vi "_RT_CtrlLoop_DigitalAnalogueInput.vi"(6 "ExpVar in":refnum<class "ExpVar.lvclass">, 8 "error in (no error)":errorcluster) -> ()   [LabVIEW 2018]
uses:
  PublicSubVI/NewExpVar/ExpVar.lvclass
  PublicSubVI/Ctl/_ctl_RT_extDO.ctl
  PublicSubVI/Ctl/_ctl_RT_FPGA_Function.ctl
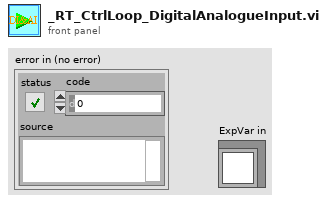
[diagram p1: front panel]
types:
  T1 = enum16{"None", "D999", "ExtAO", "ExtDO", "ExtDI_Label", "Signal_Remarks", "Script"}
  T2 = typedef "_ctl_RT_extDO.ctl" = cluster{"Label":string, "Boolean":bool}[]
  T3 = enum16{"via string label", "Laser", "Pressure", "TMP", "Script", "Signal Remarks", "ExtAO", "ExtDO", "ExtDI", "D999"}
  T4 = typedef "_ctl_RT_FPGA_Function.ctl" = enum16{"Initialisation", "Execution", "Digital In"}
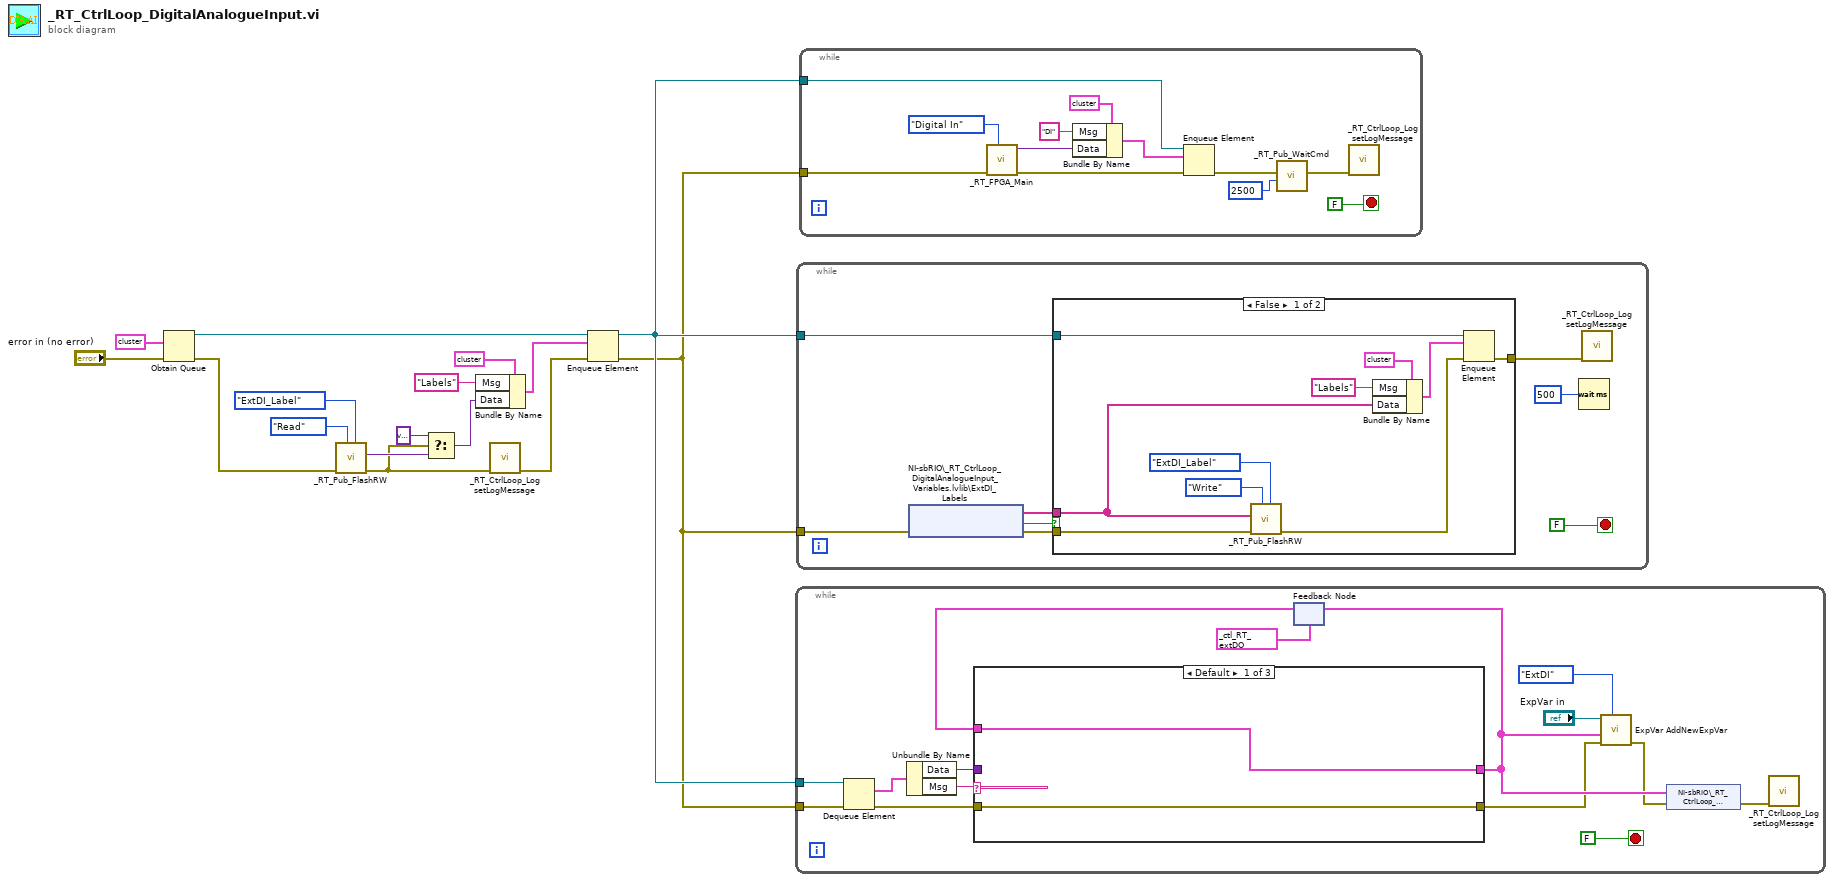
[diagram p0: block diagram]
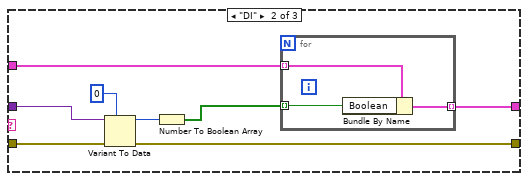
[diagram p2: hidden frame]
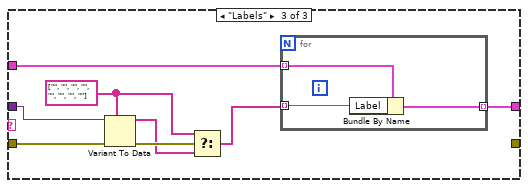
[diagram p3: hidden frame]
diagram:
  n1 = Obtain Queue(element data type=cluster{"Data":variant, "Msg":string} {"Data"=variant, "Msg"=""}, error in (no error)="error in (no error)") -> (queue out=w15:refnum<queue>, error out=w7:errorcluster)  [unwired: 3 in, 1 out]
  n2 = call "_RT_Pub_FlashRW.vi"("FileEnum"=T1."ExtDI_Label", "State"=enum16{"Read", "Write"}."Read", "error in (no error)"=w7) -> ("error out"=w2:errorcluster, "Value"=w5:variant)  [unwired: 6 in, 1 out]
  n3 = Select(t=variant, s=w2, f=w5) -> (s? t:f=w3:variant)
  n4 = Bundle By Name(cluster=cluster{"Data":variant, "Msg":string} {"Data"=variant, "Msg"=""}, "Msg"="Labels", "Data"=w3) -> (w13:cluster{"Data":variant, "Msg":string})
  n5 = call "_RT_CtrlLoop_Log setLogMessage.vi"("error in"=w2) -> ("error out"=w1:errorcluster)  [unwired: 9 in, 1 out]
  n6 = Enqueue Element(queue=w15, element=w13, error in (no error)=w1) -> (queue out=w11:refnum<queue>, error out=w10:errorcluster)  [unwired: 1 in, 1 out]
  n7 = while {
    tunnel: w11 -> [w31]
    tunnel: w10 -> [w30]
    stop <- FALSE stop-if-true
    n8 = Dequeue Element(queue=w31, error in (no error)=w30) -> (element=w19:cluster{"Data":variant, "Msg":string}, error out=w27:errorcluster)  [unwired: 1 in, 2 out]
    n9 = Unbundle By Name(w19) -> ("Data"=w28:variant, "Msg"=w29:string)
    n10 = feedback #1(T2 [{"Label"="", "Boolean"=FALSE}, {"Label"="", "Boolean"=FALSE}, {"Label"="", "Boolean"=FALSE}, {"Label"="", "Boolean"=FALSE}, {"Label"="", "Boolean"=FALSE}, {"Label"="", "Boolean"=FALSE}, {"Label"="", "Boolean"=FALSE}, {"Label"="", "Boolean"=FALSE}] ("DI in")) -> (w25:T2)
    n11 = case shown="Default" w29 {
      tunnel: w28 -> [_ w40 w52]
      tunnel: w27 -> [w32 w39 w51]
      tunnel: w25 -> [w33 w37 w50]
      tunnel: [w33 w35 w49] -> w22
      tunnel: [w32 w34 _] -> w21
      frame Default {
      }
      frame "DI" {
        n12 = Variant To Data(error in=w39, type=u8 0, Variant=w40) -> (data=w38:u8, error out=w34:errorcluster)
        n13 = Number To Boolean Array(number=w38) -> (Boolean array=w36:bool[])
        n14 = for {
          tunnel: w37 -> [w44] mode=indexing
          tunnel: w36 -> [w43] mode=indexing
          tunnel: [w42] -> w35 mode=indexing
          n15 = Bundle By Name(cluster=w44, "Boolean"=w43) -> (w42:cluster{"Label":string, "Boolean":bool})
        }
      }
      frame "Labels" {
        w46 = string[] ["", "", "", "", "", "", "", ""]
        n16 = Variant To Data(error in=w51, type=w46, Variant=w52) -> (data=w47:string[], error out=w48:errorcluster)
        n17 = Select(t=w46, s=w48, f=w47) -> (s? t:f=w45:string[])
        n18 = for {
          tunnel: w50 -> [w55] mode=indexing
          tunnel: w45 -> [w54] mode=indexing
          tunnel: [w53] -> w49 mode=indexing
          n19 = Bundle By Name(cluster=w55, "Label"=w54) -> (w53:cluster{"Label":string, "Boolean":bool})
        }
      }
    }
    n20 = feedback-in #1(w22) -> ()
    n21 = call-dynamic "ExpVar AddNewExpVar.vi"("VarType"=T3."ExtDI", "error in (no error)"=w21, "Var"=w22, "ExpVar in"="ExpVar in") -> ("error out"=w18:errorcluster)  [unwired: 6 in, 1 out]
    n22 = shared-variable "NI-sbRIO\\_RT_CtrlLoop_DigitalAnalogueInput_Variables.lvlib\\ExtDI"(w22, error in=w18) -> (error out=w17:errorcluster)
    n23 = call "_RT_CtrlLoop_Log setLogMessage.vi"("error in"=w17) -> ()  [unwired: 9 in, 2 out]
  }
  n24 = while {
    tunnel: w11 -> [w58]
    tunnel: w10 -> [w59]
    stop <- FALSE stop-if-true
    n25 = shared-variable "NI-sbRIO\\_RT_CtrlLoop_DigitalAnalogueInput_Variables.lvlib\\ExtDI_Labels"(error in=w59) -> (w60:string[], error out=w57:errorcluster, w62:bool)  [unwired: 1 in]
    n26 = case shown="False" w62 {
      tunnel: w60 -> [w68 _]
      tunnel: w58 -> [w73 _]
      tunnel: w57 -> [w67 w74]
      tunnel: [w64 w74] -> w56
      frame False {
        n27 = call "_RT_Pub_FlashRW.vi"("FileEnum"=T1."ExtDI_Label", "State"=enum16{"Read", "Write"}."Write", "error in (no error)"=w67, "DataIn"=w68) -> ("error out"=w66:errorcluster)  [unwired: 5 in, 2 out]
        n28 = Bundle By Name(cluster=cluster{"Data":variant, "Msg":string} {"Data"=variant, "Msg"=""}, "Msg"="Labels", "Data"=w68) -> (w70:cluster{"Data":variant, "Msg":string})
        n29 = Enqueue Element(queue=w73, element=w70, error in (no error)=w66) -> (error out=w64:errorcluster)  [unwired: 1 in, 2 out]
      }
      frame True {
      }
    }
    n30 = Wait (ms)(milliseconds to wait=u32 500) -> ()  [unwired: 1 out]
    n31 = call "_RT_CtrlLoop_Log setLogMessage.vi"("error in"=w56) -> ()  [unwired: 9 in, 2 out]
  }
  n32 = while {
    tunnel: w10 -> [w78]
    tunnel: w11 -> [w83]
    stop <- FALSE stop-if-true
    n33 = call "_RT_FPGA_Main.vi"("Function"=_ctl_RT_FPGA_Function."Digital In", "Error in"=w78) -> ("Error out"=w76:errorcluster, "Data out"=w80:variant)  [unwired: 7 in, 1 out]
    n34 = Bundle By Name(cluster=cluster{"Data":variant, "Msg":string} {"Data"=variant, "Msg"=""} ("element"), "Msg"="DI", "Data"=w80) -> (w81:cluster{"Data":variant, "Msg":string})
    n35 = Enqueue Element(queue=w83, element=w81, error in (no error)=w76) -> (error out=w77:errorcluster)  [unwired: 1 in, 2 out]
    n36 = call "_RT_Pub_WaitCmd.vi"("milliseconds to wait"=u32 2500, "error in (no error)"=w77) -> ("error out"=w75:errorcluster)  [unwired: 9 in]
    n37 = call "_RT_CtrlLoop_Log setLogMessage.vi"("error in"=w75) -> ()  [unwired: 9 in, 2 out]
  }
